vi "TestAnalogWrite.vi"() -> ()   [LabVIEW 2017]
uses:
  <vilib>/DAQmx/write.llb/DAQmx Write (Analog Wfm 1Chan NSamp).vi
  <vilib>/DAQmx/create/channels.llb/DAQmx Create Channel (AO-Voltage-Basic).vi
  <vilib>/DAQmx/configure/timing.llb/DAQmx Timing (Sample Clock).vi
  <vilib>/DAQmx/miscellaneous.llb/DAQmx Fill In Error Info.vi
panel:
  in  "New version":bool
  in  "physical channels":tag="PCI-DAQ/ao1"
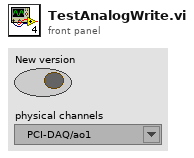
[diagram p1: front panel]
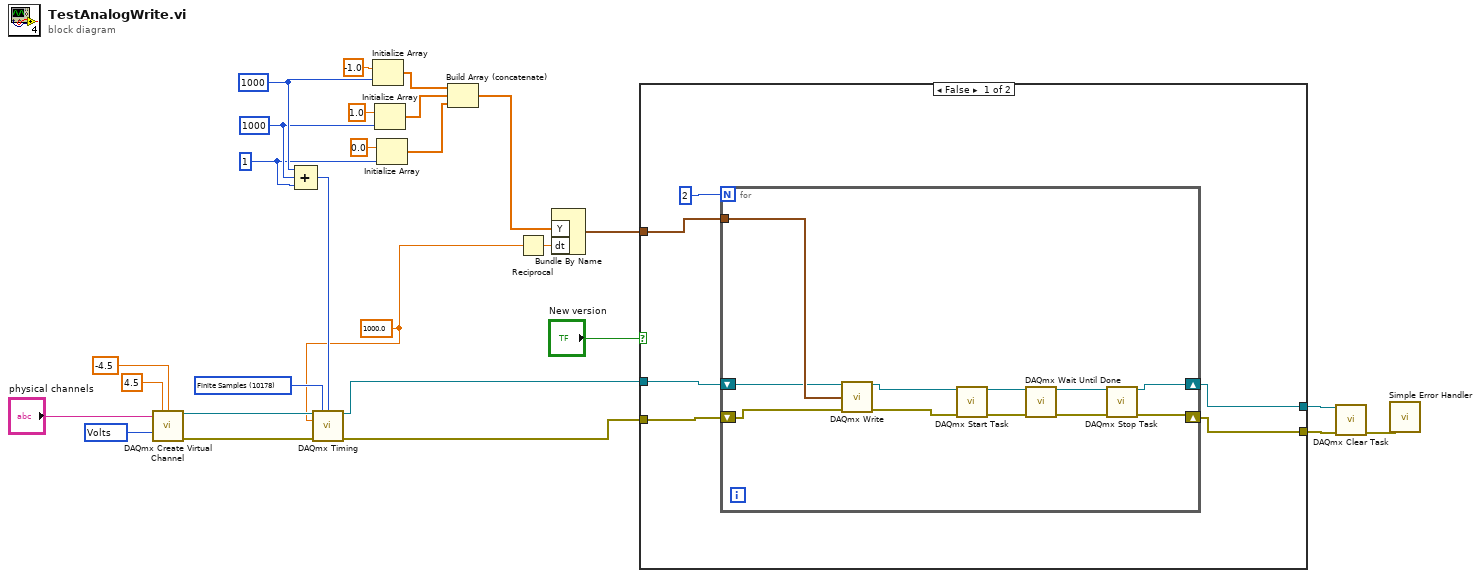
[diagram p0: block diagram]
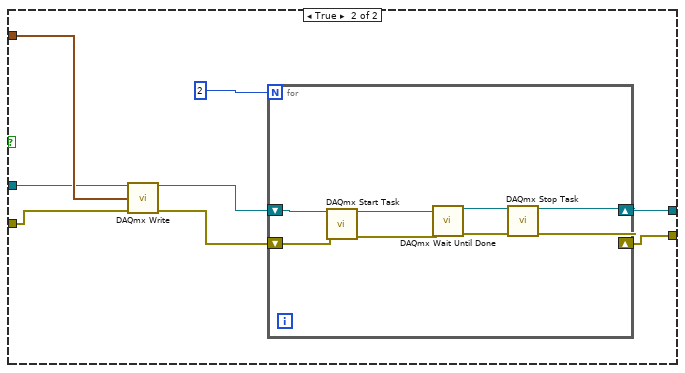
[diagram p2: hidden frame]
diagram:
  w8 = 1 ("dimension size")
  w9 = 1000 ("dimension size")
  w10 = 1000 ("dimension size")
  w21 = 10178 items=["Finite Samples"=10178, "Continuous Samples"=10123, "Hardware Timed Single Point"=12522] ("sample mode")
  w7 = 1000.0 ("rate")
  w27 = 10348 items=["Volts"=10348, "From Custom Scale"=10065] ("units")
  n1 = call-poly <vilib>:"DAQmx Create Virtual Channel.vi"("maximum value"=4.5, "minimum value"=-4.5, "physical channels"="physical channels", "units"=w27) -> ("task out"=w22:refnum<k21>, "error out"=w23:errorcluster)  [unwired: 10 in]
  n2 = Compound Arithmetic op=unknown(w10, w9, w8) -> (w11:i32)
  n3 = call-poly <vilib>:"DAQmx Timing.vi"("task/channels in"=w22, "sample mode"=w21, "samples per channel"=w11, "rate"=w7, "error in"=w23) -> ("task out"=w4:refnum<k21>, "error out"=w3:errorcluster)  [unwired: 9 in]
  n4 = Initialize Array(-1.0 ("element"), w10) -> (w14:dbl[])
  n5 = Initialize Array(1.0 ("element"), w9) -> (w18:dbl[])
  n6 = Initialize Array(0.0 ("element"), w8) -> (w12:dbl[])
  n7 = Build Array (concatenate)(w14, w18, w12) -> (w5:dbl[])
  n8 = Reciprocal(x=w7) -> (1/x=w6:dbl)
  n9 = Bundle By Name("Y"=w5, "dt"=w6) -> (w1:waveform(dbl))  [unwired: 1 in]
  n10 = case shown="False" "New version" {
    tunnel: [w33 w46] -> w17
    tunnel: [w32 w45] -> w16
    tunnel: w4 -> [w28 w50]
    tunnel: w3 -> [w29 w49]
    tunnel: w1 -> [w30 w51]
    frame False {
      n11 = for {
        N: 2 -> [_]
        shift-right: [w43] -> w32
        shift-left: w28 -> [w35]
        shift-right: [w44] -> w33
        shift-left: w29 -> [w34]
        tunnel: w30 -> [w36]
        n12 = call-poly <vilib>:"DAQmx Write.vi"("task/channels in"=w35, "data"=w36, "error in"=w34) -> ("task out"=w38:refnum<k21>, "error out"=w37:errorcluster)  [unwired: 10 in, 1 out]
        n13 = call <vilib>:"DAQmx Start Task.vi"("task/channels in"=w38, "error in"=w37) -> ("task out"=w39:refnum<k21>, "error out"=w40:errorcluster)  [unwired: 12 in]
        n14 = call <vilib>:"DAQmx Wait Until Done.vi"("task/channels in"=w39, "error in"=w40) -> ("task out"=w41:refnum<k21>, "error out"=w42:errorcluster)  [unwired: 12 in]
        n15 = call <vilib>:"DAQmx Stop Task.vi"("task/channels in"=w41, "error in"=w42) -> ("task out"=w43:refnum<k21>, "error out"=w44:errorcluster)  [unwired: 12 in]
      }
    }
    frame True {
      n16 = call-poly <vilib>:"DAQmx Write.vi"("task/channels in"=w50, "data"=w51, "error in"=w49) -> ("task out"=w47:refnum<k21>, "error out"=w48:errorcluster)  [unwired: 10 in, 1 out]
      n17 = for {
        N: 2 -> [_]
        shift-right: [w59] -> w45
        shift-left: w47 -> [w54]
        shift-right: [w60] -> w46
        shift-left: w48 -> [w53]
        n18 = call <vilib>:"DAQmx Start Task.vi"("task/channels in"=w54, "error in"=w53) -> ("task out"=w55:refnum<k21>, "error out"=w56:errorcluster)  [unwired: 12 in]
        n19 = call <vilib>:"DAQmx Wait Until Done.vi"("task/channels in"=w55, "error in"=w56) -> ("task out"=w57:refnum<k21>, "error out"=w58:errorcluster)  [unwired: 12 in]
        n20 = call <vilib>:"DAQmx Stop Task.vi"("task/channels in"=w57, "error in"=w58) -> ("task out"=w59:refnum<k21>, "error out"=w60:errorcluster)  [unwired: 12 in]
      }
    }
  }
  n21 = call <vilib>:"DAQmx Clear Task.vi"("task in"=w16, "error in"=w17) -> ("error out"=w15:errorcluster)  [unwired: 13 in]
  n22 = call <vilib>:"Simple Error Handler.vi"("error in (no error)"=w15) -> ()  [unwired: 4 in, 5 out]
